vi "Pre Launch Init.vi"(11 "Multi Instrument Handler in":refnum<class "Multi Instrument Handler.lvclass">) -> (0 "error out":errorcluster, 3 "Multi Instrument Handler out":refnum<class "Multi Instrument Handler.lvclass">)   [LabVIEW 2020, in "Instrument Handler.lvlib" / "Multi Instrument Handler.lvclass"]
doc: "(<B>Filename</B>: Actor Framework.lvlib:Actor.lvclass:Pre Launch Init.vi)\n\nDefines behavior that occurs after the Launch Nested Actor method is invoked but before the actor's Actor Core method begins running.\n\nBy default, this method does nothing. A descendant class may override it to define behavior."
uses:
  Multi Instrument Handler.lvclass
  Controls/Ctl_AquirerCompletionStatus.ctl
  Multi Instrument Handler.lvclass/Multi Instrument Handler.ctl
  PPL/HDH.Actor Framework.Core.Sequencer.lvlibp/Sequencer/Sequencer.lvclass
  Instrument Handler.lvlib
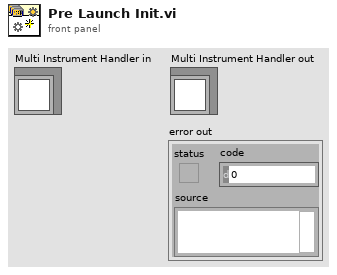
[diagram p1: front panel]
types:
  T1 = typedef "Instrument Handler.lvlib/Ctl_AquirerCompletionStatus.ctl" = cluster{"Success?":bool, "Aquirer Index":i32}
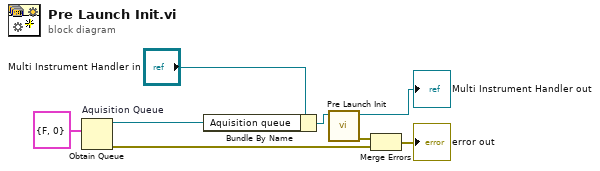
[diagram p0: block diagram]
diagram:
  n1 = Obtain Queue "Aquisition Queue"(element data type=T1 {"Success?"=FALSE, "Aquirer Index"=0} ("Instrument cluster")) -> (queue out=w3:refnum<queue>, error out=w1:errorcluster)  [unwired: 4 in, 1 out]
  n2 = Bundle By Name(cluster="Multi Instrument Handler in", "Aquisition queue"=w3) -> (w4:refnum<class "Multi Instrument Handler.lvclass">)
  n3 = call-parent "Pre Launch Init.vi"("Sequencer in"=w4) -> ("error out"=w8:errorcluster, "Sequencer out"=→"Multi Instrument Handler out":refnum<class "Multi Instrument Handler.lvclass">)  [unwired: 9 in]
  n4 = Merge Errors(w8, w1) -> (→"error out":errorcluster)
